vi "Default Configuration Parameters.vi"() -> (3 "Default Configuration":T1)   [LabVIEW 2020, in "ADAS PE Template.lvlib" / "ADAS PE Template.lvclass"]
doc: "<b>Default Configuration Parameters</b>\nThis VI allows you to define default parameter values for your plugin. These defaults will be loaded by the configuration utility when you add this plugin to a configuration."
uses:
  ADAS PE Template.lvclass
  Configuration.ctl
panel:
  # "#via_ignore"
  # "** Updates must be made on block diagram **"
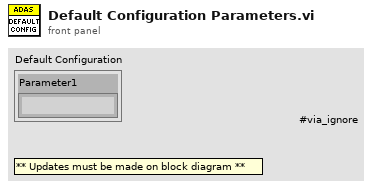
[diagram p1: front panel]
types:
  T1 = typedef "ADAS PE Template.lvlib/ADAS PE Template.lvclass/Configuration.ctl" = cluster{"Parameter1":string}
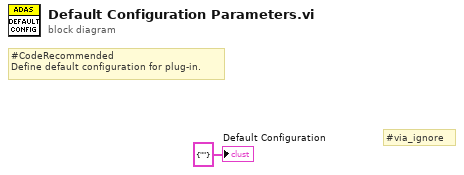
[diagram p0: block diagram]
diagram:
  # "#via_ignore"
  # "#CodeRecommended\nDefine default configuration for plug-in."
  "Default Configuration" <- T1 {"Parameter1"=""} ("Default Configuration")
